vi "PH_Sequencer.set MA Defocus Lens.vi"(0 "i ref in":refnum<vi>, 2 "Shotposition?":bool, 5 "error in":errorcluster) -> (14 "i ref out":refnum<vi>, 19 "error out":errorcluster)   [LabVIEW 2014, in "PH_Sequencer.lvlib"]
uses:
  PH_Sequencer.lvlib
  PH_Beamline/PH_Beamline.6P 4 Pos Selector Instances.ctl
  PH_4_Pos_Selector/PH_4_Pos_Selector.Position Selector.ctl
  PH_4_Pos_Selector/PH_4_Pos_Selector.lvlib
  PH_Beamline/PH_Beamline.lvlib
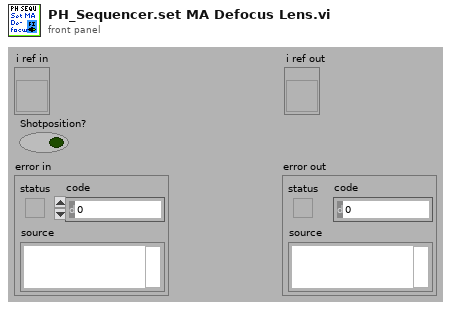
[diagram p1: front panel]
types:
  T1 = typedef "PH_Beamline.lvlib/PH_Beamline.6P 4 Pos Selector Instances.ctl" = string
  T2 = typedef "PH_4_Pos_Selector.lvlib/PH_4_Pos_Selector.Position Selector.ctl" = u16
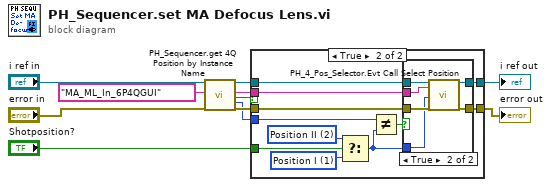
[diagram p0: block diagram]
diagram:
  n1 = call "PH_Sequencer.get 4Q Position by Instance Name.vi"("VI in"="i ref in", "Wanted 4Q Instance"=T1 "MA_ML_In_6P4QGUI", "error in"="error in") -> ("VI out"=w11:refnum<vi>, "Instancename"=w7:string, "linked"=w6:bool, "Current Position"=w5:T2, "error out"=w10:errorcluster)  [unwired: 11 in, 1 out]
  n2 = case shown="True" w6 {
    tunnel: w11 -> [w13 w24]
    tunnel: w10 -> [w12 w23]
    tunnel: w7 -> [_ w20]
    tunnel: [w13 w19] -> w9
    tunnel: [w12 w18] -> w8
    tunnel: w5 -> [_ w17]
    tunnel: "Shotposition?" -> [_ w14]
    frame False {
    }
    frame True {
      w22 = T2 1 items=["unknown", "Position I", "Position II", "Position III", "Position IV", "moving"] ("Wanted Position")
      w21 = T2 2 items=["unknown", "Position I", "Position II", "Position III", "Position IV", "moving"] ("Wanted Position")
      n3 = Select(t=w21, s=w14, f=w22) -> (s? t:f=w16:T2)
      n4 = Not Equal?(x=w17, y=w16) -> (x != y?=w15:bool)
      n5 = case shown="True" w15 {
        tunnel: w24 -> [w26 w32]
        tunnel: w23 -> [w25 w31]
        tunnel: w20 -> [_ w30]
        tunnel: [w26 w29] -> w19
        tunnel: [w25 w28] -> w18
        tunnel: w16 -> [_ w27]
        frame False {
        }
        frame True {
          n6 = call "PH_4_Pos_Selector.Evt Call Select Position.vi"("i ref in"=w32, "4 Pos instance"=w30, "Wanted Position"=w27, "error in"=w31) -> ("i ref out"=w29:refnum<vi>, "error out"=w28:errorcluster)  [unwired: 14 in]
        }
      }
    }
  }
  "i ref out" <- w9
  "error out" <- w8
